vi "IDS_MasterExample.vi"() -> ()   [LabVIEW 2016]
uses:
  VIs/Output Mode control.ctl
panel:
  out "Error 1":bool
  out "Error 3":bool
  out "IDS Status":string
  out "Error 2":bool
  in  "CLOSE":bool
  in  "Tabs":T1(tab)
  out "Connected to":string
  in  "Software Image (note: not implemented)":bool
  in  "DHCP - Server (note: not implemented)":bool
  out "ECU connected":bool
  out "ECU enabled":bool
  in  "HsslParams Input":T2
  in  "AquadB Input":T3
  in  "Environmental \nCompensation Unit":bool caption="enable ECU"
  in  "Sin-Cos Input":T4={"Period Sin-Cos and AquadB clock\n[ns]. multiple of 40ns"=40, "Resolution Sin-Cos and AquadB\n[pm/90°]"=0} {"Period Sin-Cos and AquadB clock\n[ns]. multiple of 40ns" min=40 step=40 format="%.0f ns"}
  in  "Distance Mode (not implemented)":enum16{"Absolute Position", "Displacement"}(ring)
  in  "Output Mode":T5
  in  "Master Axis (not working yet)":enum16{"Axis 1", "Axis 2", "Axis 3"}(ring)
  in  "Axis Mode":enum16{"Single Pass", "Dual Pass"}(ring)
  out "Axis 1 Contrast":cluster{i32, i32}(slide)={0, 630} caption="‰" scale=0.0..1000.0
  out "Axis 2 Contrast":cluster{i32, i32}(slide)={0, 710} caption="‰" scale=0.0..1000.0
  out "laser enabled?":bool
  in  "Enabled":bool
  out "Axis 1":string
  in  "Alignment":bool
  out "Axis 3 Contrast":cluster{i32, i32}(slide)={0, 565} caption="‰" scale=0.0..1000.0
  out "Axis 3":string
  out "Axis 2":string
  out "Axis 1 Displacement":string
  in  "Show Axis":enum16{"Axis 1", "Axis 2", "Axis 3"}(ring)
  in  "Reset Graph":bool
  out "Signalverlaufsdiagramm":dbl(graph)
  out "ECU Parameters":T6
  in  "Reset Axes":bool
  in  "Measurement":bool
  out "Axis 1":i64 caption="pm"
  out "Axis 2":i64 caption="pm"
  out "Axis 3":i64 caption="pm"
  in  "Reset Axis":bool
  in  "Milliseconds to wait":i32=10
  in  "set averageN":i32
  out "get averageN":i64
  out "Axis 2 Displacement":string
  out "Axis 3 Displacement":string
  out "Signal Quality":i32
  in  "get Info":bool
  in  "Name Device":bool
  in  "Unlock Device":bool
  in  "Lock Device":bool
  in  "Grant Access":bool
  in  "Device Name":string
  out "Info":T7
  in  "Lock by password":string
  in  "Access by password":string
  out "Grant Access Error":errorcluster
  out "Lock Error":errorcluster
  out "Unlock Error":errorcluster
  out "device Name Error":errorcluster
  out "Check Loop":errorcluster caption="Fehler (Ausgang)"
  out "ECU Loop":errorcluster
  in  "Reset Error":bool
  out "About":errorcluster
  out "Configuration":errorcluster
  out "Interface":errorcluster
  out "Alignment":errorcluster
  out "Operation":errorcluster
  out "device Handle":i32
  in  "Factory Reset":bool
  in  "Reboot System":bool
  out "Check ECU":bool
  # "Networking"
  # "Software Update"
  # "Real Time Interface"
  # "Periphery"
  # "Axis Control"
  # "Pilot Laser"
  # "Optics Alignment"
  # "Displacement"
  # "Environmental Compensation Unit"
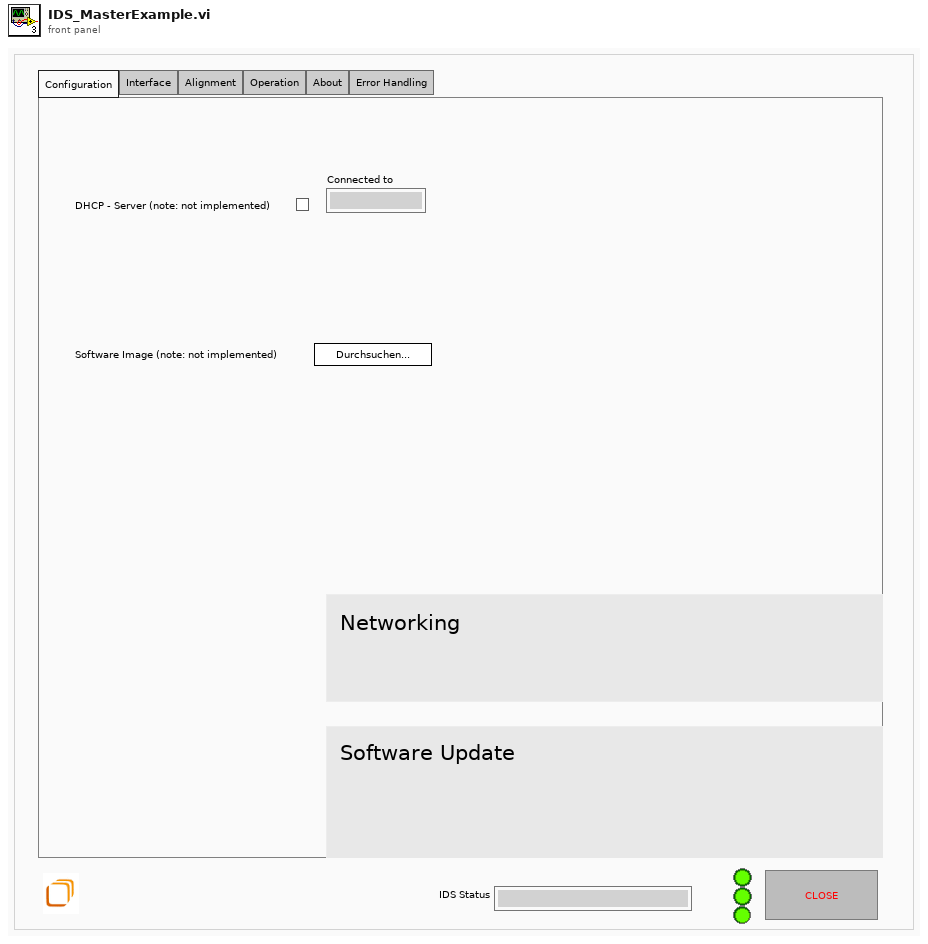
[diagram p1: front panel]
types:
  T1 = enum32{"Configuration", "Interface", "Alignment", "Operation", "About", "Error Handling"}
  T2 = cluster{"Resolution HSSL low\n2^n pm":i32, "Resolution HSSL high\n2^n pm":i32, "Period HSSL clock\n[ns]. multiple of 40ns":i32, "Period HSSL gap\n[clks]. number of clocks":i32}
  T3 = cluster{"AquadB clock\n[ns]. multiple of 40ns":dbl, "Resolution AquadB\n[pm]":dbl}
  T4 = cluster{"Period Sin-Cos and AquadB clock\n[ns]. multiple of 40ns":i32, "Resolution Sin-Cos and AquadB\n[pm/90°]":i32}
  T5 = typedef "Output Mode control.ctl" = enum16{"HSSL (LVTTL)", "HSSL (LVDS)", "AquadB (LVTTL)", "AquadB (LVDS)", "SinCos and AqudB (LVTTL Error Signal)", "SinCos and AquadB (LVDS Error Signal)"}
  T6 = cluster{"Temperature ":dbl, " Pressure":dbl, " Relative Humidity":dbl, "Refraction Index":dbl, "Status":bool}
  T7 = cluster{"Axis Signal Quality":i32, "Serial Number":string, "FPGA Version":string, "IP Adress":string, "Subnetmask":string, "Gateway":string, "dll Version":string, "Firmware version":string, "Mac Adress":string, "Device Type":string, "Device Name":string, "authorized":bool, "locked":bool}
  T8 = enum8{"Enabled", "Disabled", "Disabled and Grayed Out"}
  T9 = cluster{"IP":string, "DeviceType":string, "SerialNumber":string, "DeviceName":string, "macAddress":string, "locked":bool}[]
  T10 = cluster{"Resolution HSSL low":i32, "resolution HSSL high":i32, "HSSL Clk ":i32, "HSSL gap":i32}
  T11 = cluster{"baseline out":i32, "sn out":string, "version out":string, "addr out":string, "mask out":string, "gateway out":string, "DLL version out":string, "fw version out":string, "mac out":string, "type out":string, "name out":string, "authorized out":bool, "locked out":bool}
  T12 = cluster{"temp":dbl, "pressure":dbl, "humidity":dbl, "rIndex":dbl}
  T13 = cluster{"temp":dbl, "pressure":dbl, "humidity":dbl, "rIndex":dbl, bool}
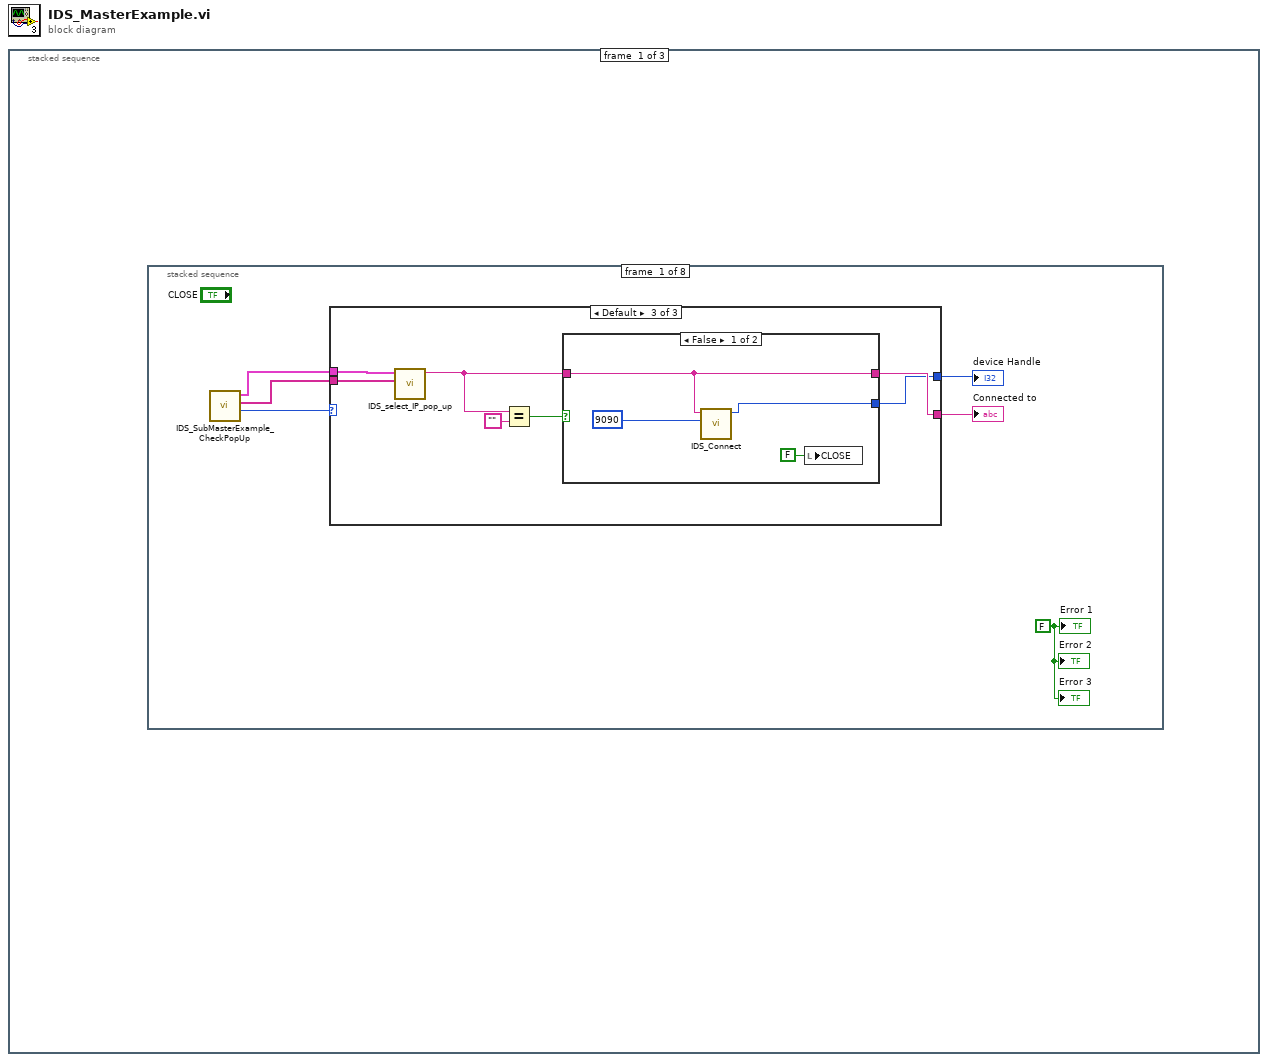
[diagram p0: block diagram]
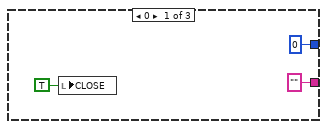
[diagram p2: hidden frame]
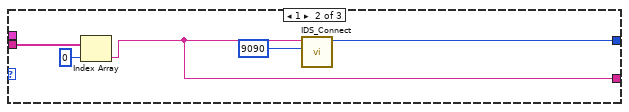
[diagram p3: hidden frame]
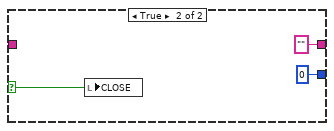
[diagram p4: hidden frame]
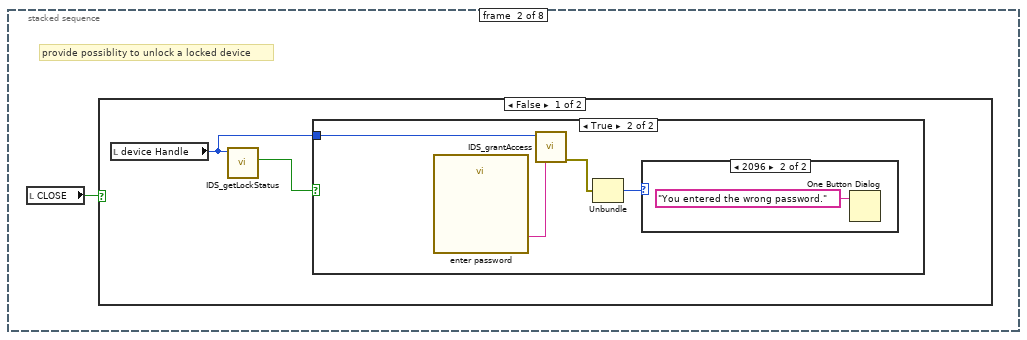
[diagram p5: hidden frame]
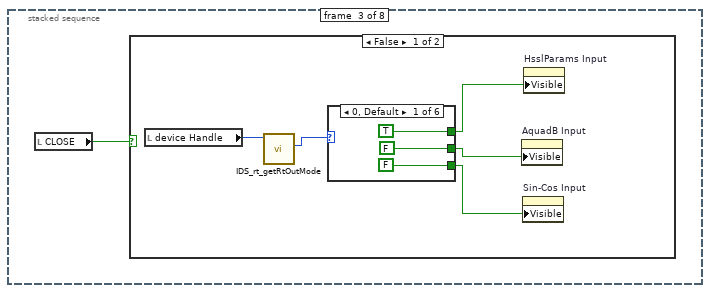
[diagram p9: hidden frame]
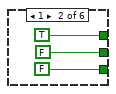
[diagram p10: hidden frame]
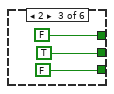
[diagram p11: hidden frame]
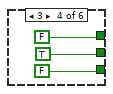
[diagram p12: hidden frame]
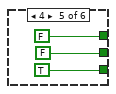
[diagram p13: hidden frame]
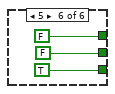
[diagram p14: hidden frame]
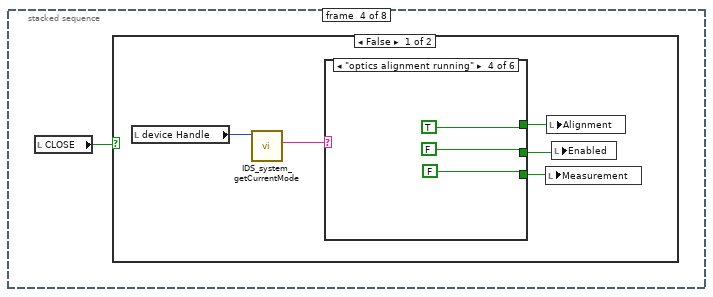
[diagram p16: hidden frame]
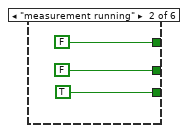
[diagram p18: hidden frame]
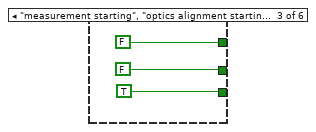
[diagram p19: hidden frame]
diagram:
  n1 = stacked-sequence {
    frame #0 {
      n2 = stacked-sequence {
        frame #0 {
          w1 = FALSE ("Error 1")
          n3 = call "IDS_SubMasterExample_CheckPopUp.vi"() -> ("No. of found devices"=w6:i32, "IPs"=w4:string[], "Found Devices"=w2:T9)  [unwired: 8 in, 1 out]
          n4 = case shown="Default" w6 {
            tunnel: [0 ("deviceHandle out") w13 w15] -> w5
            tunnel: w4 -> [_ w12 w18]
            tunnel: ["" ("IP") w10 w16] -> w3
            tunnel: w2 -> [_ _ w17]
            frame 0 {
              n5 = local write "CLOSE"(TRUE ("CLOSE")) -> ()
            }
            frame 1 {
              n6 = Index Array(array=w12, index=0) -> (element=w10:string)
              n7 = call "IDS_Connect.vi"("port"=9090, "ipAddress"=w10) -> ("deviceHandle out"=w13:i32)  [unwired: 8 in, 1 out]
            }
            frame Default {
              n8 = call "IDS_select_IP_pop_up.vi"("IPs"=w18, "Found Devices"=w17) -> ("IP"=w19:string)  [unwired: 8 in, 1 out]
              n9 = Equal?(x=w19, y="") -> (x = y?=w20:bool)
              n10 = case shown="False" w20 {
                selector: w20 -> [_ w28]
                tunnel: w19 -> [w23 _]
                tunnel: [w23 "" ("IP")] -> w16
                tunnel: [w22 0 ("deviceHandle out")] -> w15
                frame False {
                  n11 = call "IDS_Connect.vi"("port"=9090, "ipAddress"=w23) -> ("deviceHandle out"=w22:i32)  [unwired: 8 in, 1 out]
                  n12 = local write "CLOSE"(FALSE ("CLOSE")) -> ()
                }
                frame True {
                  n13 = local write "CLOSE"(w28) -> ()
                }
              }
            }
          }
          "device Handle" <- w5
          "Connected to" <- w3
          "Error 1" <- w1
          "Error 3" <- w1
          "Error 2" <- w1
        }
        frame #1 {
          # "provide possiblity to unlock a locked device"
          n14 = local read "CLOSE"() -> (w29:bool)
          n15 = case shown="False" w29 {
            frame False {
              n16 = local read "device Handle"() -> (w30:i32)
              n17 = call "IDS_getLockStatus.vi"("deviceHandle"=w30) -> ("locked out"=w31:bool)  [unwired: 7 in, 3 out]
              n18 = case shown="True" w31 {
                tunnel: w30 -> [_ w35]
                frame False {
                }
                frame True {
                  n19 = call "enter password"() -> ("password"=w34:string)  [unwired: 17 in, 2 out]
                  n20 = call "IDS_grantAccess.vi"("password"=w34, "deviceHandle"=w35) -> ("error out"=w33:errorcluster)  [unwired: 8 in, 1 out]
                  n21 = Unbundle(w33) -> ("code"=w32:i32)  [unwired: 2 out]
                  n22 = case shown="2096" w32 {
                    frame 0, Default {
                    }
                    frame 2096 {
                      n23 = One Button Dialog(message="You entered the wrong password." ("Nachricht")) -> ()  [unwired: 1 in, 1 out]
                    }
                  }
                }
              }
            }
            frame True {
            }
          }
        }
        frame #2 {
          n24 = local read "CLOSE"() -> (w37:bool)
          n25 = case shown="False" w37 {
            frame False {
              n26 = local read "device Handle"() -> (w39:i32)
              n27 = call "IDS_rt_getRtOutMode.vi"("deviceHandle"=w39) -> ("rtOutMode out"=w38:i32)  [unwired: 8 in, 2 out]
              n28 = case shown="0, Default" w38 {
                tunnel: [TRUE TRUE FALSE FALSE FALSE FALSE] -> w42
                tunnel: [FALSE FALSE TRUE TRUE FALSE FALSE] -> w41
                tunnel: [FALSE FALSE FALSE FALSE TRUE TRUE] -> w40
                frame 0, Default {
                }
                frame 1 {
                }
                frame 2 {
                }
                frame 3 {
                }
                frame 4 {
                }
                frame 5 {
                }
              }
              n29 = property on="AquadB Input" class="Clust (strict)"("Visible"=w41) -> ()  [unwired: 2 in, 2 out]
              n30 = property on="Sin-Cos Input" class="Clust (strict)"("Visible"=w40) -> ()  [unwired: 2 in, 2 out]
              n31 = property on="HsslParams Input" class="Clust (strict)"("Visible"=w42) -> ()  [unwired: 2 in, 2 out]
            }
            frame True {
            }
          }
        }
        frame #3 {
          n32 = local read "CLOSE"() -> (w61:bool)
          n33 = case shown="False" w61 {
            frame False {
              n34 = local read "device Handle"() -> (w63:i32)
              n35 = call "IDS_system_getCurrentMode.vi"("deviceHandle"=w63) -> ("mode out"=w62:string)  [unwired: 8 in, 2 out]
              n36 = case shown="\"optics alignment running\"" w62 {
                tunnel: [_ FALSE FALSE FALSE _ TRUE] -> w66
                tunnel: [_ FALSE FALSE TRUE _ FALSE] -> w65
                tunnel: [_ TRUE TRUE FALSE _ FALSE] -> w64
                frame "no change", Default {
                }
                frame "measurement running" {
                }
                frame "measurement starting", "optics alignment starting" {
                }
                frame "optics alignment running" {
                }
                frame "system idle" {
                }
                frame "pilot laser enabled" {
                }
              }
              n37 = local write "Measurement"(w64) -> ()
              n38 = local write "Alignment"(w65) -> ()
              n39 = local write "Enabled"(w66) -> ()
            }
            frame True {
            }
          }
        }
        frame #4 {
          n40 = local read "CLOSE"() -> (w79:bool)
          n41 = case shown="False" w79 {
            frame False {
              n42 = local read "device Handle"() -> (w81:i32)
              n43 = call "IDS_axis_getPassMode.vi"("deviceHandle"=w81) -> ("mode out"=w80:i32)  [unwired: 8 in, 2 out]
              n44 = local write "Axis Mode"(w80) -> ()
              n45 = local write "get Info"(TRUE ("get Info")) -> ()
            }
            frame True {
            }
          }
        }
        frame #5 {
          n46 = local read "CLOSE"() -> (w83:bool)
          n47 = case shown="False" w83 {
            frame False {
              w84 = T8."Enabled" ("Deaktiviert")
              n48 = property on="AquadB Input" class="Clust (strict)"("DisabledEnum"=w84) -> ()  [unwired: 2 in, 2 out]
              n49 = property on="Sin-Cos Input" class="Clust (strict)"("DisabledEnum"=w84) -> ()  [unwired: 2 in, 2 out]
              n50 = property on="Output Mode" class="Enum (strict)"("DisabledEnum"=w84) -> ()  [unwired: 2 in, 2 out]
              n51 = property on="HsslParams Input" class="Clust (strict)"("DisabledEnum"=w84) -> ()  [unwired: 2 in, 2 out]
              n52 = property on="Master Axis (not working yet)" class="Enum (strict)"("DisabledEnum"=w84) -> ()  [unwired: 2 in, 2 out]
              n53 = property on="Alignment" class="Bool (strict)"("DisabledEnum"=w84) -> ()  [unwired: 2 in, 2 out]
              n54 = property on="Enabled" class="Bool (strict)"("DisabledEnum"=w84) -> ()  [unwired: 2 in, 2 out]
              n55 = property on="Measurement" class="Bool (strict)"("DisabledEnum"=w84) -> ()  [unwired: 2 in, 2 out]
              n56 = property on="Distance Mode (not implemented)" class="Enum (strict)"("DisabledEnum"=w84) -> ()  [unwired: 2 in, 2 out]
              n57 = property on="Axis Mode" class="Enum (strict)"("DisabledEnum"=w84) -> ()  [unwired: 2 in, 2 out]
            }
            frame True {
            }
          }
        }
        frame #6 {
          n58 = local read "CLOSE"() -> (w85:bool)
          n59 = case shown="False" w85 {
            frame False {
              n60 = control-ref of="Axis 3"() -> (w92:refnum<vi>)
              n61 = control-ref of="Axis 1"() -> (w97:refnum<vi>)
              n62 = control-ref of="Axis 2"() -> (w93:refnum<vi>)
              n63 = property class="Str"(reference=w97, "Visible"=FALSE) -> ()  [unwired: 1 in, 2 out]
              n64 = property class="Str"(reference=w93, "Visible"=FALSE) -> ()  [unwired: 1 in, 2 out]
              n65 = property class="Str"(reference=w92, "Visible"=FALSE) -> ()  [unwired: 1 in, 2 out]
              n66 = control-ref of="Axis 1 Displacement"() -> (w88:refnum<vi>)
              n67 = control-ref of="Axis 2 Displacement"() -> (w87:refnum<vi>)
              n68 = control-ref of="Axis 3 Displacement"() -> (w86:refnum<vi>)
              n69 = property class="Str"(reference=w86, "Visible"=FALSE) -> ()  [unwired: 1 in, 2 out]
              n70 = property class="Str"(reference=w88, "Visible"=FALSE) -> ()  [unwired: 1 in, 2 out]
              n71 = property class="Str"(reference=w87, "Visible"=FALSE) -> ()  [unwired: 1 in, 2 out]
            }
            frame True {
            }
          }
        }
        frame #7 {
          # "Init"
          n72 = local read "CLOSE"() -> (w98:bool)
          n73 = case shown="False" w98 {
            frame False {
              w99 = FALSE ("ECU enabled")
              w100 = i64 0 ("Axis 3")
              w102 = cluster{i32, i32} {0, 0} ("Axis 1 Contrast")
              n74 = local write "ECU enabled"(w99) -> ()
              n75 = local write "Axis 1 Contrast"(w102) -> ()
              n76 = local write "Axis 2 Contrast"(w102) -> ()
              n77 = local write "Axis 3 Contrast"(w102) -> ()
              n78 = local write "ECU Parameters"(T6 {"Temperature "=0.0, " Pressure"=0.0, " Relative Humidity"=0.0, "Refraction Index"=0.0, "Status"=FALSE} ("ECU Parameters")) -> ()
              n79 = local write "Axis 3"(w100) -> ()
              n80 = local write "Axis 2"(w100) -> ()
              n81 = local write "Axis 1"(w100) -> ()
              n82 = local write "Signal Quality"(w100) -> ()
              n83 = local write "ECU connected"(w99) -> ()
            }
            frame True {
            }
          }
        }
      }
    }
    frame #1 {
      n84 = local read "CLOSE"() -> (w103:bool)
      n85 = case shown="False" w103 {
        frame False {
          n86 = while {
            shift-right: [w107] -> _
            shift-left: _ -> [w112]
            shift-right: [w105] -> _
            shift-left: _ -> [w108]
            stop <- w109 stop-if-true
            # "Status Check Loop"
            n87 = local read "device Handle"() -> (w106:i32)
            n88 = Wait (ms)(milliseconds to wait=u32 500) -> ()  [unwired: 1 out]
            n89 = call "IDS_system_getCurrentMode.vi"("error in (no error)"=w108, "deviceHandle"=w106) -> ("error out"=w105:errorcluster, "mode out"=w107:string)  [unwired: 7 in, 1 out]
            "IDS Status" <- w107
            n90 = Equal?(x=w112, y=w107) -> (x = y?=w113:bool)
            n91 = Select(t="no change", s=w113, f=w107) -> (s? t:f=w114:string)
            n92 = case shown="\"measurement starting\"" w114 {
              tunnel: [FALSE TRUE FALSE FALSE FALSE FALSE FALSE] -> w111
              frame "no change", Default {
              }
              frame "measurement running" {
                w118 = T8."Disabled and Grayed Out" ("Deaktiviert")
                n93 = local write "Measurement"(TRUE ("Measurement")) -> ()
                n94 = local write "Alignment"(FALSE ("Alignment")) -> ()
                n95 = local write "Enabled"(FALSE ("Enabled")) -> ()
                n96 = property on="AquadB Input" class="Clust (strict)"("DisabledEnum"=w118) -> ()  [unwired: 2 in, 2 out]
                n97 = property on="Sin-Cos Input" class="Clust (strict)"("DisabledEnum"=w118) -> ()  [unwired: 2 in, 2 out]
                n98 = property on="Output Mode" class="Enum (strict)"("DisabledEnum"=w118) -> ()  [unwired: 2 in, 2 out]
                n99 = property on="HsslParams Input" class="Clust (strict)"("DisabledEnum"=w118) -> ()  [unwired: 2 in, 2 out]
                n100 = property on="Master Axis (not working yet)" class="Enum (strict)"("DisabledEnum"=w118) -> ()  [unwired: 2 in, 2 out]
                n101 = property on="Alignment" class="Bool (strict)"("DisabledEnum"=w118) -> ()  [unwired: 2 in, 2 out]
                n102 = property on="Enabled" class="Bool (strict)"("DisabledEnum"=w118) -> ()  [unwired: 2 in, 2 out]
                n103 = property on="Measurement" class="Bool (strict)"("DisabledEnum"=T8."Enabled" ("Deaktiviert")) -> ()  [unwired: 2 in, 2 out]
                n104 = property on="Distance Mode" class="Enum (strict)"("DisabledEnum"=w118) -> ()  [unwired: 2 in, 2 out]
                n105 = property on="Axis Mode" class="Enum (strict)"("DisabledEnum"=w118) -> ()  [unwired: 2 in, 2 out]
              }
              frame "measurement starting" {
                n106 = stacked-sequence {
                  frame #0 {
                    w124 = T8."Disabled and Grayed Out" ("Deaktiviert")
                    n107 = local write "Measurement"(TRUE ("Measurement")) -> ()
                    n108 = local write "Alignment"(FALSE ("Alignment")) -> ()
                    n109 = local write "Enabled"(FALSE ("Enabled")) -> ()
                    n110 = property on="Sin-Cos Input" class="Clust (strict)"("DisabledEnum"=w124) -> ()  [unwired: 2 in, 2 out]
                    n111 = property on="Output Mode" class="Enum (strict)"("DisabledEnum"=w124) -> ()  [unwired: 2 in, 2 out]
                    n112 = property on="Master Axis (not working yet)" class="Enum (strict)"("DisabledEnum"=w124) -> ()  [unwired: 2 in, 2 out]
                    n113 = property on="Alignment" class="Bool (strict)"("DisabledEnum"=w124) -> ()  [unwired: 2 in, 2 out]
                    n114 = property on="Enabled" class="Bool (strict)"("DisabledEnum"=w124) -> ()  [unwired: 2 in, 2 out]
                    n115 = property on="Measurement" class="Bool (strict)"("DisabledEnum"=w124) -> ()  [unwired: 2 in, 2 out]
                    n116 = property on="AquadB Input" class="Clust (strict)"("DisabledEnum"=w124) -> ()  [unwired: 2 in, 2 out]
                    n117 = property on="HsslParams Input" class="Clust (strict)"("DisabledEnum"=w124) -> ()  [unwired: 2 in, 2 out]
                    n118 = property on="Distance Mode" class="Enum (strict)"("DisabledEnum"=w124) -> ()  [unwired: 2 in, 2 out]
                    n119 = property on="Axis Mode" class="Enum (strict)"("DisabledEnum"=w124) -> ()  [unwired: 2 in, 2 out]
                  }
                }
              }
              frame "optics alignment starting" {
                n120 = stacked-sequence {
                  frame #0 {
                    w129 = T8."Disabled and Grayed Out" ("Deaktiviert")
                    n121 = local write "Measurement"(TRUE ("Measurement")) -> ()
                    n122 = local write "Alignment"(FALSE ("Alignment")) -> ()
                    n123 = local write "Enabled"(FALSE ("Enabled")) -> ()
                    n124 = property on="Sin-Cos Input" class="Clust (strict)"("DisabledEnum"=w129) -> ()  [unwired: 2 in, 2 out]
                    n125 = property on="Output Mode" class="Enum (strict)"("DisabledEnum"=w129) -> ()  [unwired: 2 in, 2 out]
                    n126 = property on="Master Axis (not working yet)" class="Enum (strict)"("DisabledEnum"=w129) -> ()  [unwired: 2 in, 2 out]
                    n127 = property on="Alignment" class="Bool (strict)"("DisabledEnum"=w129) -> ()  [unwired: 2 in, 2 out]
                    n128 = property on="Enabled" class="Bool (strict)"("DisabledEnum"=w129) -> ()  [unwired: 2 in, 2 out]
                    n129 = property on="Measurement" class="Bool (strict)"("DisabledEnum"=w129) -> ()  [unwired: 2 in, 2 out]
                    n130 = property on="AquadB Input" class="Clust (strict)"("DisabledEnum"=w129) -> ()  [unwired: 2 in, 2 out]
                    n131 = property on="HsslParams Input" class="Clust (strict)"("DisabledEnum"=w129) -> ()  [unwired: 2 in, 2 out]
                    n132 = property on="Distance Mode" class="Enum (strict)"("DisabledEnum"=w129) -> ()  [unwired: 2 in, 2 out]
                    n133 = property on="Axis Mode" class="Enum (strict)"("DisabledEnum"=w129) -> ()  [unwired: 2 in, 2 out]
                  }
                }
              }
              frame "optics alignment running" {
                w134 = T8."Disabled and Grayed Out" ("Deaktiviert")
                n134 = local write "Measurement"(FALSE ("Measurement")) -> ()
                n135 = local write "Alignment"(TRUE ("Alignment")) -> ()
                n136 = local write "Enabled"(FALSE ("Enabled")) -> ()
                n137 = property on="AquadB Input" class="Clust (strict)"("DisabledEnum"=w134) -> ()  [unwired: 2 in, 2 out]
                n138 = property on="Sin-Cos Input" class="Clust (strict)"("DisabledEnum"=w134) -> ()  [unwired: 2 in, 2 out]
                n139 = property on="Output Mode" class="Enum (strict)"("DisabledEnum"=w134) -> ()  [unwired: 2 in, 2 out]
                n140 = property on="HsslParams Input" class="Clust (strict)"("DisabledEnum"=w134) -> ()  [unwired: 2 in, 2 out]
                n141 = property on="Master Axis (not working yet)" class="Enum (strict)"("DisabledEnum"=w134) -> ()  [unwired: 2 in, 2 out]
                n142 = property on="Alignment" class="Bool (strict)"("DisabledEnum"=T8."Enabled" ("Deaktiviert")) -> ()  [unwired: 2 in, 2 out]
                n143 = property on="Enabled" class="Bool (strict)"("DisabledEnum"=w134) -> ()  [unwired: 2 in, 2 out]
                n144 = property on="Measurement" class="Bool (strict)"("DisabledEnum"=w134) -> ()  [unwired: 2 in, 2 out]
                n145 = property on="Distance Mode" class="Enum (strict)"("DisabledEnum"=w134) -> ()  [unwired: 2 in, 2 out]
                n146 = property on="Axis Mode" class="Enum (strict)"("DisabledEnum"=w134) -> ()  [unwired: 2 in, 2 out]
              }
              frame "system idle" {
                w139 = T8."Enabled" ("Deaktiviert")
                n147 = property on="AquadB Input" class="Clust (strict)"("DisabledEnum"=w139) -> ()  [unwired: 2 in, 2 out]
                n148 = property on="Sin-Cos Input" class="Clust (strict)"("DisabledEnum"=w139) -> ()  [unwired: 2 in, 2 out]
                n149 = property on="Output Mode" class="Enum (strict)"("DisabledEnum"=w139) -> ()  [unwired: 2 in, 2 out]
                n150 = property on="HsslParams Input" class="Clust (strict)"("DisabledEnum"=w139) -> ()  [unwired: 2 in, 2 out]
                n151 = property on="Master Axis (not working yet)" class="Enum (strict)"("DisabledEnum"=w139) -> ()  [unwired: 2 in, 2 out]
                n152 = property on="Alignment" class="Bool (strict)"("DisabledEnum"=w139) -> ()  [unwired: 2 in, 2 out]
                n153 = property on="Enabled" class="Bool (strict)"("DisabledEnum"=w139) -> ()  [unwired: 2 in, 2 out]
                n154 = property on="Measurement" class="Bool (strict)"("DisabledEnum"=w139) -> ()  [unwired: 2 in, 2 out]
                n155 = property on="Distance Mode" class="Enum (strict)"("DisabledEnum"=w139) -> ()  [unwired: 2 in, 2 out]
                n156 = property on="Axis Mode" class="Enum (strict)"("DisabledEnum"=w139) -> ()  [unwired: 2 in, 2 out]
              }
              frame "pilot laser enabled" {
                w142 = T8."Disabled and Grayed Out" ("Deaktiviert")
                n157 = local write "Measurement"(FALSE ("Measurement")) -> ()
                n158 = local write "Alignment"(FALSE ("Alignment")) -> ()
                n159 = local write "Enabled"(TRUE ("Enabled")) -> ()
                n160 = property on="AquadB Input" class="Clust (strict)"("DisabledEnum"=w142) -> ()  [unwired: 2 in, 2 out]
                n161 = property on="Sin-Cos Input" class="Clust (strict)"("DisabledEnum"=w142) -> ()  [unwired: 2 in, 2 out]
                n162 = property on="Output Mode" class="Enum (strict)"("DisabledEnum"=w142) -> ()  [unwired: 2 in, 2 out]
                n163 = property on="HsslParams Input" class="Clust (strict)"("DisabledEnum"=w142) -> ()  [unwired: 2 in, 2 out]
                n164 = property on="Master Axis (not working yet)" class="Enum (strict)"("DisabledEnum"=w142) -> ()  [unwired: 2 in, 2 out]
                n165 = property on="Alignment" class="Bool (strict)"("DisabledEnum"=w142) -> ()  [unwired: 2 in, 2 out]
                n166 = property on="Enabled" class="Bool (strict)"("DisabledEnum"=T8."Enabled" ("Deaktiviert")) -> ()  [unwired: 2 in, 2 out]
                n167 = property on="Measurement" class="Bool (strict)"("DisabledEnum"=w142) -> ()  [unwired: 2 in, 2 out]
                n168 = property on="Distance Mode" class="Enum (strict)"("DisabledEnum"=w142) -> ()  [unwired: 2 in, 2 out]
                n169 = property on="Axis Mode" class="Enum (strict)"("DisabledEnum"=w142) -> ()  [unwired: 2 in, 2 out]
              }
            }
            "Check ECU" <- w111
            n170 = Unbundle By Name(w105) -> ("status"=w104:bool)
            n171 = local read "CLOSE"() -> (w109:bool)
            n172 = local write "Error 1"(w104) -> ()
          }
          n173 = while {
            shift-right: [w179] -> _
            shift-left: _ -> [w180]
            stop <- w176 stop-if-true
            # "Event / Tab Loop"
            n174 = local read "device Handle"() -> (w178:i32)
            n175 = case shown="\"About\"" "Tabs" {
              tunnel: [w182 w188 w264 w406 w503 w566] -> w179
              tunnel: w180 -> [w183 w189 w263 w405 w504 w567]
              tunnel: w178 -> [_ w187 w262 w403 w502 w565]
              frame "Configuration" {
                n176 = event shown="[0] Timeout" {
                  selector: _ -> [_ _]
                  dyn-events: _ -> [_ _]
                  timeout: 10 -> [_ _]
                  tunnel: [w185 w186] -> w182
                  tunnel: w183 -> [w185 w186]
                  event Timeout {
                    n177 = event-data() -> ()  [unwired: 1 in, 1 out]
                  }
                  event "DHCP - Server (note: not implemented)", "Software Image (note: not implemented)": Value Change {
                    n178 = event-data() -> ()  [unwired: 1 in, 1 out]
                  }
                }
                "Configuration" <- w182
              }
              frame "Interface" {
                n179 = event shown="[0] \"HsslParams Input\": Value Change" {
                  selector: _ -> [_ _ _ _ _ _ _]
                  dyn-events: _ -> [_ _ _ _ _ _ _]
                  timeout: 10 -> [_ _ _ _ _ _ _]
                  tunnel: [w194 w214 w219 w224 w227 w241 w261] -> w188
                  tunnel: w189 -> [w195 w215 w220 w225 w228 w242 w261]
                  tunnel: w187 -> [w191 w207 w217 w222 w226 w237 _]
                  event "HsslParams Input": Value Change {
                    n180 = event-data() -> ()  [unwired: 1 in, 1 out]
                    n181 = local read "HsslParams Input"() -> (w192:T2)
                    n182 = call "IDS_rt_ParametersHssl.vi"("Error In"=w195, "set?"=TRUE ("Read write"), "HsslParams Input"=w192, "deviceHandle"=w191) -> ("Error Out"=w194:errorcluster)  [unwired: 5 in, 2 out]
                  }
                  event Timeout {
                    n183 = event-data() -> ()  [unwired: 1 in, 1 out]
                    n184 = call "IDS_rt_getRtOutMode.vi"("error in (no error)"=w215, "deviceHandle"=w207) -> ("error out"=w212:errorcluster, "deviceHandle out"=w206:i32)  [unwired: 7 in, 1 out]
                    n185 = call "IDS_rt_getPeriodSinCosClk.vi"("error in (no error)"=w212, "deviceHandle"=w206) -> ("error out"=w197:errorcluster, "period out"=w205:i32, "deviceHandle out"=w196:i32)  [unwired: 7 in]
                    n186 = call "IDS_rt_get_ResolutionSinCos.vi"("error in (no error)"=w197, "deviceHandle"=w196) -> ("error out"=w208:errorcluster, "resolution out"=w204:i32, "deviceHandle out"=w203:i32)  [unwired: 7 in]
                    n187 = Bundle("period out"=w205, "resolution out"=w204) -> (w213:cluster{"period out":i32, "resolution out":i32})  [unwired: 1 in]
                    n188 = local write "Sin-Cos Input"(w213) -> ()
                    n189 = call "IDS_rt_ParametersHssl.vi"("Error In"=w208, "set?"=FALSE ("Read write"), "deviceHandle"=w203) -> ("Error Out"=w210:errorcluster, "HsslParams Output"=w198:T10, "deviceHandle out"=w202:i32)  [unwired: 6 in]
                    n190 = local write "HsslParams Input"(w198) -> ()
                    n191 = call "IDS_ecu_isEnabled.vi"("error in (no error)"=w210, "deviceHandle"=w202) -> ("error out"=w211:errorcluster, "enabled out"=→"ECU enabled":bool, "deviceHandle out"=w201:i32)  [unwired: 7 in]
                    n192 = call "IDS_ecu_isConnected.vi"("error in (no error)"=w211, "deviceHandle"=w201) -> ("error out"=w214:errorcluster, "connected out"=→"ECU connected":bool)  [unwired: 7 in, 1 out]
                  }
                  event "Sin-Cos Input.Period Sin-Cos and AquadB clock\n[ns]. multiple of 40ns": Value Change {
                    n193 = event-data() -> ()  [unwired: 1 in, 1 out]
                    n194 = local read "Sin-Cos Input"() -> (w218:T4)
                    n195 = Unbundle(w218) -> ("Period Sin-Cos and AquadB clock\n[ns]. multiple of 40ns"=w216:i32)  [unwired: 1 out]
                    n196 = call "IDS_rt_setPeriodSinCosClk.vi"("error in (no error)"=w220, "period"=w216, "deviceHandle"=w217) -> ("error out"=w219:errorcluster)  [unwired: 7 in, 1 out]
                  }
                  event "Sin-Cos Input.Resolution Sin-Cos and AquadB\n[pm/90°]": Value Change {
                    n197 = event-data() -> ()  [unwired: 1 in, 1 out]
                    n198 = local read "Sin-Cos Input"() -> (w223:T4)
                    n199 = Unbundle(w223) -> ("Resolution Sin-Cos and AquadB\n[pm/90°]"=w221:i32)  [unwired: 1 out]
                    n200 = call "IDS_rt_setResolutionSinCos.vi"("error in (no error)"=w225, "resolution"=w221, "deviceHandle"=w222) -> ("error out"=w224:errorcluster)  [unwired: 7 in, 1 out]
                  }
                  event "Environmental \nCompensation Unit": Value Change {
                    n201 = event-data() -> ()  [unwired: 1 in, 1 out]
                    n202 = case shown="True" "Environmental \nCompensation Unit" {
                      tunnel: w228 -> [w232 w235]
                      tunnel: [w231 w234] -> w227
                      tunnel: w226 -> [w230 w233]
                      frame False {
                        n203 = call "IDS_ecu_disable.vi"("error in (no error)"=w232, "deviceHandle"=w230) -> ("error out"=w231:errorcluster)  [unwired: 8 in, 1 out]
                      }
                      frame True {
                        n204 = call "IDS_ecu_enable.vi"("error in (no error)"=w235, "deviceHandle"=w233) -> ("error out"=w234:errorcluster)  [unwired: 8 in, 1 out]
                      }
                    }
                  }
                  event Value Change {
                    n205 = event-data() -> ()  [unwired: 1 in, 1 out]
                    n206 = call "IDS_rt_setRtOutMode.vi"("error in (no error)"=w242, "rtOutMode"="Output Mode", "deviceHandle"=w237) -> ("error out"=w241:errorcluster)  [unwired: 7 in, 1 out]
                    n207 = case shown="\"SinCos and AquadB (LVDS Error Signal)\"" "Output Mode" {
                      tunnel: [TRUE TRUE FALSE FALSE FALSE FALSE] -> w240
                      tunnel: [FALSE FALSE TRUE TRUE FALSE FALSE] -> w239
                      tunnel: [FALSE FALSE FALSE FALSE TRUE TRUE] -> w238
                      frame "HSSL (LVTTL)", Default {
                      }
                      frame "HSSL (LVDS)" {
                      }
                      frame "AquadB (LVTTL)" {
                      }
                      frame "AquadB (LVDS)" {
                      }
                      frame "SinCos and AqudB (LVTTL Error Signal)" {
                      }
                      frame "SinCos and AquadB (LVDS Error Signal)" {
                      }
                    }
                    n208 = property on="HsslParams Input" class="Clust (strict)"("Visible"=w240) -> ()  [unwired: 2 in, 2 out]
                    n209 = property on="AquadB Input" class="Clust (strict)"("Visible"=w239) -> ()  [unwired: 2 in, 2 out]
                    n210 = property on="Sin-Cos Input" class="Clust (strict)"("Visible"=w238) -> ()  [unwired: 2 in, 2 out]
                  }
                  event "Distance Mode (not implemented)": Value Change {
                    n211 = event-data() -> ()  [unwired: 1 in, 1 out]
                  }
                }
                "Interface" <- w188
              }
              frame "Alignment", Default {
                n212 = event shown="[0] Timeout" {
                  selector: _ -> [_ _ _ _]
                  dyn-events: _ -> [_ _ _ _]
                  timeout: 10 -> [_ _ _ _]
                  tunnel: w263 -> [w270 w373 w391 w402]
                  tunnel: [w271 w372 w390 w401] -> w264
                  tunnel: w262 -> [w266 w371 w389 w400]
                  event Timeout {
                    n213 = event-data() -> ()  [unwired: 1 in, 1 out]
                    n214 = local read "IDS Status"() -> (w269:string)
                    n215 = Equal?(x=w269, y="optics alignment running") -> (x = y?=w268:bool)
                    n216 = case shown="True" w268 {
                      tunnel: [w277 _] -> w271
                      tunnel: w270 -> [w272 w285]
                      tunnel: w266 -> [w276 w286]
                      frame False {
                        n217 = control-ref of="Axis 2"() -> (w280:refnum<vi>)
                        n218 = control-ref of="Axis 3"() -> (w281:refnum<vi>)
                        n219 = control-ref of="Axis 1"() -> (w279:refnum<vi>)
                        n220 = property class="Str"(reference=w279, "Visible"=FALSE) -> ()  [unwired: 1 in, 2 out]
                        n221 = property class="Str"(reference=w280, "Visible"=FALSE) -> ()  [unwired: 1 in, 2 out]
                        n222 = property class="Str"(reference=w281, "Visible"=FALSE) -> ()  [unwired: 1 in, 2 out]
                        n223 = call "IDS_axis_getPassMode.vi"("error in (no error)"=w272, "deviceHandle"=w276) -> ("error out"=w278:errorcluster, "mode out"=w274:i32, "deviceHandle out"=w275:i32)  [unwired: 7 in]
                        n224 = call "IDS_laser_isEnabled.vi"("error in (no error)"=w278, "deviceHandle"=w275) -> ("error out"=w277:errorcluster, "enabled out"=→"laser enabled?":bool)  [unwired: 7 in, 1 out]
                        n225 = local write "Axis Mode"(w274) -> ()
                      }
                      frame True {
                        n226 = stacked-sequence {
                          tunnel: w285 -> [w301 _ _ _]
                          tunnel: w286 -> [w300 _ _ _]
                          frame #0 {
                            n227 = call "IDS_adjustment_getContrastInPermill.vi"("deviceHandle"=w300, "axisNumber"=1, "error in (no error)"=w301) -> ("contrast out"=w293:i32, "baseline out"=w292:i32, "error out"=w306:errorcluster)  [unwired: 8 in, 2 out]
                            n228 = call "IDS_adjustment_getContrastInPermill.vi"("deviceHandle"=w300, "axisNumber"=0, "error in (no error)"=w301) -> ("contrast out"=w291:i32, "baseline out"=w290:i32, "error out"=w307:errorcluster)  [unwired: 8 in, 2 out]
                            n229 = call "IDS_adjustment_getContrastInPermill.vi"("deviceHandle"=w300, "axisNumber"=2, "error in (no error)"=w301) -> ("contrast out"=w296:i32, "baseline out"=w295:i32, "error out"=w287:errorcluster)  [unwired: 8 in, 2 out]
                            n230 = Bundle("contrast out"=w293, "baseline out"=w292) -> (→"Axis 2 Contrast":cluster{"contrast out":i32, "baseline out":i32})  [unwired: 1 in]
                            n231 = Bundle("contrast out"=w291, "baseline out"=w290) -> (→"Axis 1 Contrast":cluster{"contrast out":i32, "baseline out":i32})  [unwired: 1 in]
                            n232 = Bundle("contrast out"=w296, "baseline out"=w295) -> (→"Axis 3 Contrast":cluster{"contrast out":i32, "baseline out":i32})  [unwired: 1 in]
                            n233 = control-ref of="Axis 1"() -> (w304:refnum<vi>)
                            n234 = control-ref of="Axis 2"() -> (w303:refnum<vi>)
                            n235 = control-ref of="Axis 3"() -> (w302:refnum<vi>)
                            n236 = Build Array(w307, w306, w287) -> (w305:errorcluster[])
                            n237 = call "IDS_SubMasterExample_ErrorMessages.vi"("String in 1"=w304, "String in 2"=w303, "String in 3"=w302, "appended array"=w305) -> ()  [unwired: 16 in]
                          }
                          frame #1 {
                            n238 = local read "Axis 1 Contrast"() -> (w312:cluster{i32, i32})
                            n239 = Unbundle(w312) -> (w311:i32)  [unwired: 1 out]
                            n240 = In Range and Coerce(upper limit=250.0, x=w311, lower limit=0.0) -> (In Range?=w310:bool)  [unwired: 1 out]
                            n241 = In Range and Coerce(upper limit=500.0, x=w311, lower limit=250.0) -> (In Range?=w309:bool)  [unwired: 1 out]
                            n242 = In Range and Coerce(upper limit=750.0, x=w311, lower limit=500.0) -> (In Range?=w308:bool)  [unwired: 1 out]
                            n243 = case shown="False" w310 {
                              tunnel: [w322 u32 15663104] -> w319
                              tunnel: w309 -> [w321 _]
                              tunnel: w308 -> [w320 _]
                              frame False {
                                n244 = case shown="False" w321 {
                                tunnel: [w324 u32 15705600] -> w322
                                tunnel: w320 -> [w323 _]
                                frame False {
                                n245 = case shown="True" w323 {
                                tunnel: [u32 1634048 u32 12386114] -> w324
                                frame False {
                                }
                                frame True {
                                }
                                }
                                }
                                frame True {
                                }
                                }
                              }
                              frame True {
                              }
                            }
                            n246 = property on="Axis 1 Contrast" class="Slide (strict)"("Fill Color"=w319) -> ()  [unwired: 2 in, 2 out]
                          }
                          frame #2 {
                            n247 = local read "Axis 2 Contrast"() -> (w333:cluster{i32, i32})
                            n248 = Unbundle(w333) -> (w332:i32)  [unwired: 1 out]
                            n249 = In Range and Coerce(upper limit=250.0, x=w332, lower limit=0.0) -> (In Range?=w331:bool)  [unwired: 1 out]
                            n250 = In Range and Coerce(upper limit=500.0, x=w332, lower limit=250.0) -> (In Range?=w330:bool)  [unwired: 1 out]
                            n251 = In Range and Coerce(upper limit=750.0, x=w332, lower limit=500.0) -> (In Range?=w329:bool)  [unwired: 1 out]
                            n252 = case shown="False" w331 {
                              tunnel: [w343 u32 15663104] -> w340
                              tunnel: w330 -> [w342 _]
                              tunnel: w329 -> [w341 _]
                              frame False {
                                n253 = case shown="False" w342 {
                                tunnel: [w345 u32 15705600] -> w343
                                tunnel: w341 -> [w344 _]
                                frame False {
                                n254 = case shown="False" w344 {
                                tunnel: [u32 1634048 u32 12386114] -> w345
                                frame False {
                                }
                                frame True {
                                }
                                }
                                }
                                frame True {
                                }
                                }
                              }
                              frame True {
                              }
                            }
                            n255 = property on="Axis 2 Contrast" class="Slide (strict)"("Fill Color"=w340) -> ()  [unwired: 2 in, 2 out]
                          }
                          frame #3 {
                            n256 = local read "Axis 3 Contrast"() -> (w354:cluster{i32, i32})
                            n257 = Unbundle(w354) -> (w353:i32)  [unwired: 1 out]
                            n258 = In Range and Coerce(upper limit=250.0, x=w353, lower limit=0.0) -> (In Range?=w352:bool)  [unwired: 1 out]
                            n259 = In Range and Coerce(upper limit=500.0, x=w353, lower limit=250.0) -> (In Range?=w351:bool)  [unwired: 1 out]
                            n260 = In Range and Coerce(upper limit=750.0, x=w353, lower limit=500.0) -> (In Range?=w350:bool)  [unwired: 1 out]
                            n261 = case shown="False" w352 {
                              tunnel: [w364 u32 15663104] -> w361
                              tunnel: w351 -> [w363 _]
                              tunnel: w350 -> [w362 _]
                              frame False {
                                n262 = case shown="False" w363 {
                                tunnel: [w366 u32 15705600] -> w364
                                tunnel: w362 -> [w365 _]
                                frame False {
                                n263 = case shown="False" w365 {
                                tunnel: [u32 1634048 u32 12386114] -> w366
                                frame False {
                                }
                                frame True {
                                }
                                }
                                }
                                frame True {
                                }
                                }
                              }
                              frame True {
                              }
                            }
                            n264 = property on="Axis 3 Contrast" class="Slide (strict)"("Fill Color"=w361) -> ()  [unwired: 2 in, 2 out]
                          }
                        }
                      }
                    }
                  }
                  event "Alignment": Value Change {
                    n265 = event-data() -> ()  [unwired: 1 in, 1 out]
                    n266 = case shown="False" "Alignment" {
                      tunnel: w373 -> [w384 w388]
                      tunnel: [w383 w387] -> w372
                      tunnel: w371 -> [w376 w386]
                      frame False {
                        w375 = cluster{i32, i32} {0, 0} ("Axis 1 Contrast")
                        n267 = call "IDS_system_stopOpticsAlignment.vi"("error in (no error)"=w384, "deviceHandle"=w376) -> ("error out"=w383:errorcluster)  [unwired: 8 in, 1 out]
                        n268 = control-ref of="Axis 1"() -> (w380:refnum<vi>)
                        n269 = control-ref of="Axis 2"() -> (w381:refnum<vi>)
                        n270 = control-ref of="Axis 3"() -> (w382:refnum<vi>)
                        n271 = property class="Str"(reference=w380, "Visible"=FALSE) -> ()  [unwired: 1 in, 2 out]
                        n272 = property class="Str"(reference=w381, "Visible"=FALSE) -> ()  [unwired: 1 in, 2 out]
                        n273 = property class="Str"(reference=w382, "Visible"=FALSE) -> ()  [unwired: 1 in, 2 out]
                        n274 = local write "Axis 1 Contrast"(w375) -> ()
                        n275 = local write "Axis 3 Contrast"(w375) -> ()
                        n276 = local write "Axis 2 Contrast"(w375) -> ()
                      }
                      frame True {
                        w385 = cluster{i32, i32} {0, 0} ("Axis 1 Contrast")
                        n277 = call "IDS_system_startOpticsAlignment.vi"("error in (no error)"=w388, "deviceHandle"=w386) -> ("error out"=w387:errorcluster)  [unwired: 8 in, 1 out]
                        n278 = local write "Axis 1 Contrast"(w385) -> ()
                        n279 = local write "Axis 2 Contrast"(w385) -> ()
                        n280 = local write "Axis 3 Contrast"(w385) -> ()
                      }
                    }
                  }
                  event "Enabled": Value Change {
                    n281 = event-data() -> ()  [unwired: 1 in, 1 out]
                    n282 = case shown="True" "Enabled" {
                      tunnel: w391 -> [w395 w398]
                      tunnel: [w394 w397] -> w390
                      tunnel: w389 -> [w393 w396]
                      frame False {
                        n283 = call "IDS_laser_disable.vi"("error in (no error)"=w395, "deviceHandle"=w393) -> ("error out"=w394:errorcluster)  [unwired: 8 in, 1 out]
                      }
                      frame True {
                        n284 = call "IDS_laser_enable.vi"("error in (no error)"=w398, "deviceHandle"=w396) -> ("error out"=w397:errorcluster)  [unwired: 8 in, 1 out]
                      }
                    }
                  }
                  event "Axis Mode", "Master Axis (not working yet)": Value Change {
                    n285 = event-data() -> ()  [unwired: 1 in, 1 out]
                    n286 = call "IDS_axis_setPassMode.vi"("error in (no error)"=w402, "mode"="Axis Mode", "deviceHandle"=w400) -> ("error out"=w401:errorcluster)  [unwired: 7 in, 1 out]
                  }
                }
                "Alignment" <- w264
              }
              frame "Operation" {
                n287 = event shown="[0] Timeout" {
                  selector: _ -> [_ _ _ _ _ _]
                  dyn-events: _ -> [_ _ _ _ _ _]
                  timeout: "Milliseconds to wait" -> [_ _ _ _ _ _]
                  tunnel: [w412 w463 w480 w489 w496 w500] -> w406
                  tunnel: w405 -> [w411 w464 w481 w490 w496 w501]
                  tunnel: w403 -> [w407 w456 w478 w488 _ w498]
                  event Timeout {
                    n288 = event-data() -> ()  [unwired: 1 in, 1 out]
                    n289 = local read "IDS Status"() -> (w409:string)
                    n290 = Equal?(x=w409, y="measurement running") -> (x = y?=w410:bool)
                    n291 = case shown="True" w410 {
                      tunnel: [w414 _] -> w412
                      tunnel: w411 -> [w414 w416]
                      tunnel: w407 -> [_ w415]
                      frame False {
                        n292 = local write "get Info"(TRUE ("get Info")) -> ()
                      }
                      frame True {
                        n293 = stacked-sequence {
                          tunnel: w416 -> [w429 w438 w441 _]
                          tunnel: w415 -> [w419 w434 w439 w442]
                          frame #0 {
                            n294 = call "IDS_displacement_getAxesDisplacement.vi"("deviceHandle"=w419, "error in (no error)"=w429) -> ("deviceHandle out"=w418:i32, "disp axis 1"=w421:i64, "disp axis 2"=w417:i64, "disp axis 3"=w428:i64, "error out"=w422:errorcluster)  [unwired: 9 in]
                            n295 = call "IDS_displacement_getAbsolutePositions.vi"("deviceHandle"=w418, "error in (no error)"=w422) -> ("position axis 1"=w425:i64, "position axis 2"=w424:i64, "position axis 3"=w423:i64)  [unwired: 9 in, 2 out]
                            n296 = Add(x=w421, y=w425) -> (x+y=→"Axis 1":i64)
                            n297 = Add(x=w417, y=w424) -> (x+y=→"Axis 2":i64)
                            n298 = Add(x=w428, y=w423) -> (x+y=→"Axis 3":i64)
                          }
                          frame #1 {
                            n299 = call "IDS_displacement_getAxisDisplacement.vi"("error in (no error)"=w438, "axis"="Show Axis", "deviceHandle"=w434) -> ("error out"=w433:errorcluster, "displacement"=w435:i64, "deviceHandle out"=w431:i32)  [unwired: 6 in]
                            n300 = call "IDS_system_getAxisSignalQuality.vi"("deviceHandle"=w431, "axisNumber"="Show Axis", "error in (no error)"=w433) -> ("baseline out"=→"Signal Quality":i32)  [unwired: 4 in, 3 out]
                            n301 = Divide(x=w435, y=i64 1000000) -> (x/y=→"Signalverlaufsdiagramm":dbl)
                          }
                          frame #2 {
                            n302 = call "IDS_displacement_getAverageN.vi"("error in (no error)"=w441, "deviceHandle"=w439) -> ("averageN out"=→"get averageN":i64)  [unwired: 7 in, 2 out]
                          }
                          frame #3 {
                            n303 = local read "get Info"() -> (w443:bool)
                            n304 = case shown="True" w443 {
                              tunnel: w442 -> [_ w447]
                              frame False {
                              }
                              frame True {
                                n305 = local write "get Info"(FALSE) -> ()
                                n306 = call "IDS_displacement_getAbsolutePosition.vi"("axis"=0, "deviceHandle"=w447) -> ("error out"=w455:errorcluster)  [unwired: 7 in, 2 out]
                                n307 = call "IDS_displacement_getAbsolutePosition.vi"("axis"=1, "deviceHandle"=w447) -> ("error out"=w454:errorcluster)  [unwired: 7 in, 2 out]
                                n308 = call "IDS_displacement_getAbsolutePosition.vi"("axis"=2, "deviceHandle"=w447) -> ("error out"=w453:errorcluster)  [unwired: 7 in, 2 out]
                                n309 = control-ref of="Axis 1 Displacement"() -> (w451:refnum<vi>)
                                n310 = Build Array(w455, w454, w453) -> (w452:errorcluster[])
                                n311 = control-ref of="Axis 2 Displacement"() -> (w450:refnum<vi>)
                                n312 = control-ref of="Axis 3 Displacement"() -> (w449:refnum<vi>)
                                n313 = call "IDS_SubMasterExample_ErrorMessages.vi"("String in 1"=w451, "String in 2"=w450, "String in 3"=w449, "appended array"=w452) -> ()  [unwired: 16 in]
                              }
                            }
                          }
                        }
                      }
                    }
                  }
                  event "Measurement": Value Change {
                    n314 = event-data() -> ()  [unwired: 1 in, 1 out]
                    n315 = control-ref of="Axis 1 Displacement"() -> (w461:refnum<vi>)
                    n316 = control-ref of="Axis 3 Displacement"() -> (w457:refnum<vi>)
                    n317 = control-ref of="Axis 2 Displacement"() -> (w458:refnum<vi>)
                    n318 = property class="Str"(reference=w461, "Visible"=FALSE) -> ()  [unwired: 1 in, 2 out]
                    n319 = property class="Str"(reference=w458, "Visible"=FALSE) -> ()  [unwired: 1 in, 2 out]
                    n320 = property class="Str"(reference=w457, "Visible"=FALSE) -> ()  [unwired: 1 in, 2 out]
                    n321 = case shown="False" "Measurement" {
                      tunnel: w464 -> [w471 w477]
                      tunnel: [w470 w476] -> w463
                      tunnel: w456 -> [w466 w472]
                      frame False {
                        n322 = call "IDS_system_stopMeasurement.vi"("error in (no error)"=w471, "deviceHandle"=w466) -> ("error out"=w470:errorcluster)  [unwired: 8 in, 1 out]
                        n323 = local write "Axis 2"(i64 0 ("Axis 2")) -> ()
                        n324 = local write "Axis 1"(i64 0 ("Axis 1")) -> ()
                        n325 = local write "Axis 3"(i64 0 ("Axis 3")) -> ()
                      }
                      frame True {
                        n326 = call "IDS_system_startMeasurement.vi"("error in (no error)"=w477, "deviceHandle"=w472) -> ("error out"=w476:errorcluster)  [unwired: 8 in, 1 out]
                        n327 = local write "Axis 2"(i64 0 ("Axis 2")) -> ()
                        n328 = local write "Axis 1"(i64 0 ("Axis 1")) -> ()
                        n329 = local write "Axis 3"(i64 0 ("Axis 3")) -> ()
                      }
                    }
                  }
                  event "Reset Axis": Value Change {
                    n330 = event-data() -> ()  [unwired: 1 in, 1 out]
                    n331 = local read "Show Axis"() -> (w479:enum16{"Axis 1", "Axis 2", "Axis 3"})
                    n332 = case shown="True" "Reset Axis" {
                      tunnel: w481 -> [w483 w487]
                      tunnel: [w483 w486] -> w480
                      tunnel: w479 -> [_ w485]
                      tunnel: w478 -> [_ w484]
                      frame False {
                      }
                      frame True {
                        n333 = call "IDS_system_resetAxis.vi"("error in (no error)"=w487, "axis"=w485, "deviceHandle"=w484) -> ("error out"=w486:errorcluster)  [unwired: 7 in, 1 out]
                      }
                    }
                  }
                  event "Reset Axes": Value Change {
                    n334 = event-data() -> ()  [unwired: 1 in, 1 out]
                    n335 = case shown="True" "Reset Axes" {
                      tunnel: w490 -> [w492 w494]
                      tunnel: [w492 w493] -> w489
                      tunnel: w488 -> [_ w495]
                      frame False {
                      }
                      frame True {
                        n336 = call "IDS_system_resetAxes.vi"("error in (no error)"=w494, "deviceHandle"=w495) -> ("error out"=w493:errorcluster)  [unwired: 8 in, 1 out]
                      }
                    }
                  }
                  event "Reset Graph": Value Change {
                    # "Reset Graph"
                    n337 = event-data() -> ()  [unwired: 1 in, 1 out]
                    n338 = property on="Signalverlaufsdiagramm" class="WFChart (strict)"("History Data"=i32[] []) -> ()  [unwired: 2 in, 2 out]
                  }
                  event "set averageN": Value Change {
                    n339 = event-data() -> ()  [unwired: 1 in, 1 out]
                    n340 = call "IDS_displacement_setAverageN.vi"("error in (no error)"=w501, "averageN"="set averageN", "deviceHandle"=w498) -> ("error out"=w500:errorcluster)  [unwired: 7 in, 1 out]
                  }
                }
                "Operation" <- w406
              }
              frame "About" {
                n341 = event shown="[0] Timeout" {
                  selector: _ -> [_ _ _ _ _]
                  dyn-events: _ -> [_ _ _ _ _]
                  timeout: u32 100 ("milliseconds to wait") -> [_ _ _ _ _]
                  tunnel: w504 -> [w527 w548 w553 w559 w563]
                  tunnel: [w528 errorcluster {"status"=FALSE, "code"=0, "source"=""} ("error out") errorcluster {"status"=FALSE, "code"=0, "source"=""} ("error out") errorcluster {"status"=FALSE, "code"=0, "source"=""} ("error out") errorcluster {"status"=FALSE, "code"=0, "source"=""} ("error out")] -> w503
                  tunnel: w502 -> [w545 w549 w555 w560 w564]
                  event Timeout {
                    n342 = event-data() -> ()  [unwired: 1 in, 1 out]
                    n343 = call "IDS_system_getAxisSignalQuality.vi"("deviceHandle"=w545, "axisNumber"=0, "error in (no error)"=w527) -> ("deviceHandle out"=w524:i32, "baseline out"=w539:i32, "error out"=w519:errorcluster)  [unwired: 4 in, 1 out]
                    n344 = call "IDS_system_getSerialNumber.vi"("error in (no error)"=w519, "deviceHandle"=w524) -> ("error out"=w518:errorcluster, "sn out"=w538:string, "deviceHandle out"=w523:i32)  [unwired: 7 in]
                    n345 = call "IDS_system_getFpgaVersion.vi"("error in (no error)"=w518, "deviceHandle"=w523) -> ("error out"=w517:errorcluster, "version out"=w537:string, "deviceHandle out"=w522:i32)  [unwired: 7 in]
                    n346 = call "IDS_system_getIpAddress.vi"("error in (no error)"=w517, "deviceHandle"=w522) -> ("error out"=w516:errorcluster, "addr out"=w536:string, "deviceHandle out"=w521:i32)  [unwired: 7 in]
                    n347 = call "IDS_system_getSubnetMask.vi"("error in (no error)"=w516, "deviceHandle"=w521) -> ("error out"=w515:errorcluster, "mask out"=w535:string, "deviceHandle out"=w520:i32)  [unwired: 7 in]
                    n348 = call "IDS_system_getGateway.vi"("error in (no error)"=w515, "deviceHandle"=w520) -> ("error out"=w510:errorcluster, "gateway out"=w534:string, "deviceHandle out"=w544:i32)  [unwired: 7 in]
                    n349 = call "IDS_GetDllVersion.vi"("error in (no error)"=w510, "deviceHandle"=w544) -> ("error out"=w509:errorcluster, "DLL version out"=w533:string, "deviceHandle out"=w543:i32)  [unwired: 7 in]
                    n350 = call "IDS_system_getFirmwareVersion.vi"("error in (no error)"=w509, "deviceHandle"=w543) -> ("error out"=w512:errorcluster, "fw version out"=w506:string, "deviceHandle out"=w514:i32)  [unwired: 7 in]
                    n351 = call "IDS_system_getMacAddress.vi"("error in (no error)"=w512, "deviceHandle"=w514) -> ("error out"=w511:errorcluster, "mac out"=w532:string, "deviceHandle out"=w513:i32)  [unwired: 7 in]
                    n352 = call "IDS_system_getDeviceType.vi"("error in (no error)"=w511, "deviceHandle"=w513) -> ("error out"=w526:errorcluster, "type out"=w531:string, "deviceHandle out"=w542:i32)  [unwired: 7 in]
                    n353 = call "IDS_system_getDeviceName.vi"("deviceHandle"=w542, "error in (no error)"=w526) -> ("deviceHandle out"=w541:i32, "name out"=w530:string, "error out"=w525:errorcluster)  [unwired: 6 in]
                    n354 = call "IDS_getLockStatus.vi"("error in (no error)"=w525, "deviceHandle"=w541) -> ("error out"=w528:errorcluster, "authorized out"=w507:bool, "locked out"=w508:bool)  [unwired: 6 in, 1 out]
                    n355 = Bundle("baseline out"=w539, "sn out"=w538, "version out"=w537, "addr out"=w536, "mask out"=w535, "gateway out"=w534, "DLL version out"=w533, "fw version out"=w506, "mac out"=w532, "type out"=w531, "name out"=w530, "authorized out"=w507, "locked out"=w508) -> (→"Info":T11)  [unwired: 1 in]
                  }
                  event "Name Device": Value Change {
                    n356 = event-data() -> ()  [unwired: 1 in, 3 out]
                    n357 = call "IDS_system_setDeviceName.vi"("error in (no error)"=w548, "name"="Device Name", "deviceHandle"=w549) -> ("error out"=→"device Name Error":errorcluster)  [unwired: 7 in, 1 out]
                  }
                  event "Grant Access": Value Change {
                    n358 = event-data() -> ()  [unwired: 1 in, 1 out]
                    n359 = call "IDS_grantAccess.vi"("error in (no error)"=w553, "password"="Access by password", "deviceHandle"=w555) -> ("error out"=→"Grant Access Error":errorcluster)  [unwired: 7 in, 1 out]
                  }
                  event "Lock Device": Value Change {
                    n360 = event-data() -> ()  [unwired: 1 in, 6 out]
                    n361 = call "IDS_lock.vi"("error in (no error)"=w559, "password"="Lock by password", "deviceHandle"=w560) -> ("error out"=→"Lock Error":errorcluster)  [unwired: 7 in, 1 out]
                  }
                  event "Unlock Device": Value Change {
                    n362 = event-data() -> ()  [unwired: 1 in, 1 out]
                    n363 = call "IDS_unlock.vi"("error in (no error)"=w563, "deviceHandle"=w564) -> ("error out"=→"Unlock Error":errorcluster)  [unwired: 8 in, 1 out]
                  }
                }
                "About" <- w503
              }
              frame "Error Handling" {
                n364 = event shown="[3] \"Reboot System\": Value Change" {
                  selector: _ -> [_ _ _ _]
                  dyn-events: _ -> [_ _ _ _]
                  timeout: 500 -> [_ _ _ _]
                  tunnel: w567 -> [w569 w571 w574 w576]
                  tunnel: [w569 w570 w573 w575] -> w566
                  tunnel: w565 -> [_ w572 _ _]
                  event Timeout {
                    n365 = event-data() -> ()  [unwired: 1 in, 1 out]
                  }
                  event "Reset Error": Value Change {
                    n366 = event-data() -> ()  [unwired: 1 in, 1 out]
                    n367 = call "IDS_system_resetError.vi"("error in (no error)"=w571, "deviceHandle"=w572) -> ("error out"=w570:errorcluster)  [unwired: 8 in, 1 out]
                  }
                  event "Factory Reset": Value Change {
                    n368 = event-data() -> ()  [unwired: 1 in, 1 out]
                    n369 = call "IDS_system_factoryReset.vi"("error in (no error)"=w574) -> ("error out"=w573:errorcluster)  [unwired: 9 in, 1 out]
                  }
                  event "Reboot System": Value Change {
                    n370 = event-data() -> ()  [unwired: 1 in, 1 out]
                    n371 = call "IDS_system_rebootSystem.vi"("error in (no error)"=w576) -> ("error out"=w575:errorcluster)  [unwired: 9 in, 1 out]
                  }
                }
              }
            }
            n372 = local read "CLOSE"() -> (w176:bool)
            n373 = Unbundle By Name(w179) -> ("status"=w177:bool)
            n374 = local write "Error 2"(w177) -> ()
          }
          n375 = while {
            shift-right: [w148] -> _
            shift-left: _ -> [w150]
            stop <- w153 stop-if-true
            # "ECU Data"
            n376 = local read "device Handle"() -> (w149:i32)
            n377 = local read "Check ECU"() -> (w152:bool)
            n378 = Wait (ms)(milliseconds to wait=u32 500) -> ()  [unwired: 1 out]
            n379 = case shown="False" w152 {
              tunnel: [w154 w162] -> w148
              tunnel: w150 -> [w154 w161]
              tunnel: w149 -> [_ w159]
              frame False {
              }
              frame True {
                n380 = call "IDS_ecu_isEnabled.vi"("error in (no error)"=w161, "deviceHandle"=w159) -> ("error out"=w163:errorcluster, "enabled out"=w157:bool, "deviceHandle out"=w158:i32)  [unwired: 7 in]
                n381 = call "IDS_ecu_isConnected.vi"("error in (no error)"=w163, "deviceHandle"=w158) -> ("error out"=w160:errorcluster, "connected out"=w156:bool, "deviceHandle out"=w155:i32)  [unwired: 7 in]
                n382 = And(x=w157, y=w156) -> (x .and. y?=w164:bool)
                n383 = case shown="True" w164 {
                  selector: w164 -> [_ w167]
                  tunnel: [w165 w174] -> w162
                  tunnel: w160 -> [w165 w175]
                  tunnel: w155 -> [_ w173]
                  frame False {
                  }
                  frame True {
                    n384 = call "IDS_ecu_getParameters.vi"("error in (no error)"=w175, "deviceHandle"=w173) -> ("error out"=w174:errorcluster, "ECU parameters"=w172:T12)  [unwired: 7 in, 1 out]
                    n385 = Unbundle(w172) -> ("temp"=w171:dbl, "pressure"=w170:dbl, "humidity"=w169:dbl, "rIndex"=w168:dbl)
                    n386 = Bundle("temp"=w171, "pressure"=w170, "humidity"=w169, "rIndex"=w168, w167) -> (→"ECU Parameters":T13)  [unwired: 1 in]
                  }
                }
              }
            }
            "ECU Loop" <- w148
            n387 = Unbundle By Name(w148) -> ("status"=w147:bool)
            n388 = local read "CLOSE"() -> (w153:bool)
            n389 = local write "Error 3"(w147) -> ()
          }
        }
        frame True {
        }
      }
    }
    frame #2 {
      n390 = stacked-sequence {
        frame #0 {
          n391 = local write "CLOSE"(FALSE ("Stopp 2")) -> ()
          n392 = local read "device Handle"() -> (w577:i32)
          n393 = call "IDS_Disconnect.vi"("deviceHandle"=w577) -> ()  [unwired: 10 in, 1 out]
        }
      }
    }
  }
